vi "Periodic Tasks.vi"(8 "error in":errorcluster) -> ()   [LabVIEW 2016]
doc: "This VI runs in parallel to other tasks. It can contain as many user-defined periodic loops as you need. These can carry out PID or other sorts of timed response."
uses:
  <vilib>/Rock Robotics/WPI/Utilities/WPI_GetSetVariantRefNum.vi
  <vilib>/Rock Robotics/Network Tables/NT Write Number.vi
  <vilib>/Instr/_visa.llb/VISA Configure Serial Port (Instr).vi
  2_11_17/Systems/Global 1.vi
panel:
  out "PSI":dbl=101.0986199
  out "Drive R0 Effort":dbl format="%#_13g"
  out "Drive L0 Effort":dbl format="%#_13g"
  out "read buffer":string="B:2,X:203.00"
  in  "Search_Params":string[](array[string])=["B", "X", "Y", "W1", "H1", "W2", "H2"]
  out "Last Complete Message":string="B:2,X:203.00,Y:125.00,W1:11,H1:27,W2:8,H2:25"
  out "length":i32=44
  in  "off set":dbl format="%#_13g"
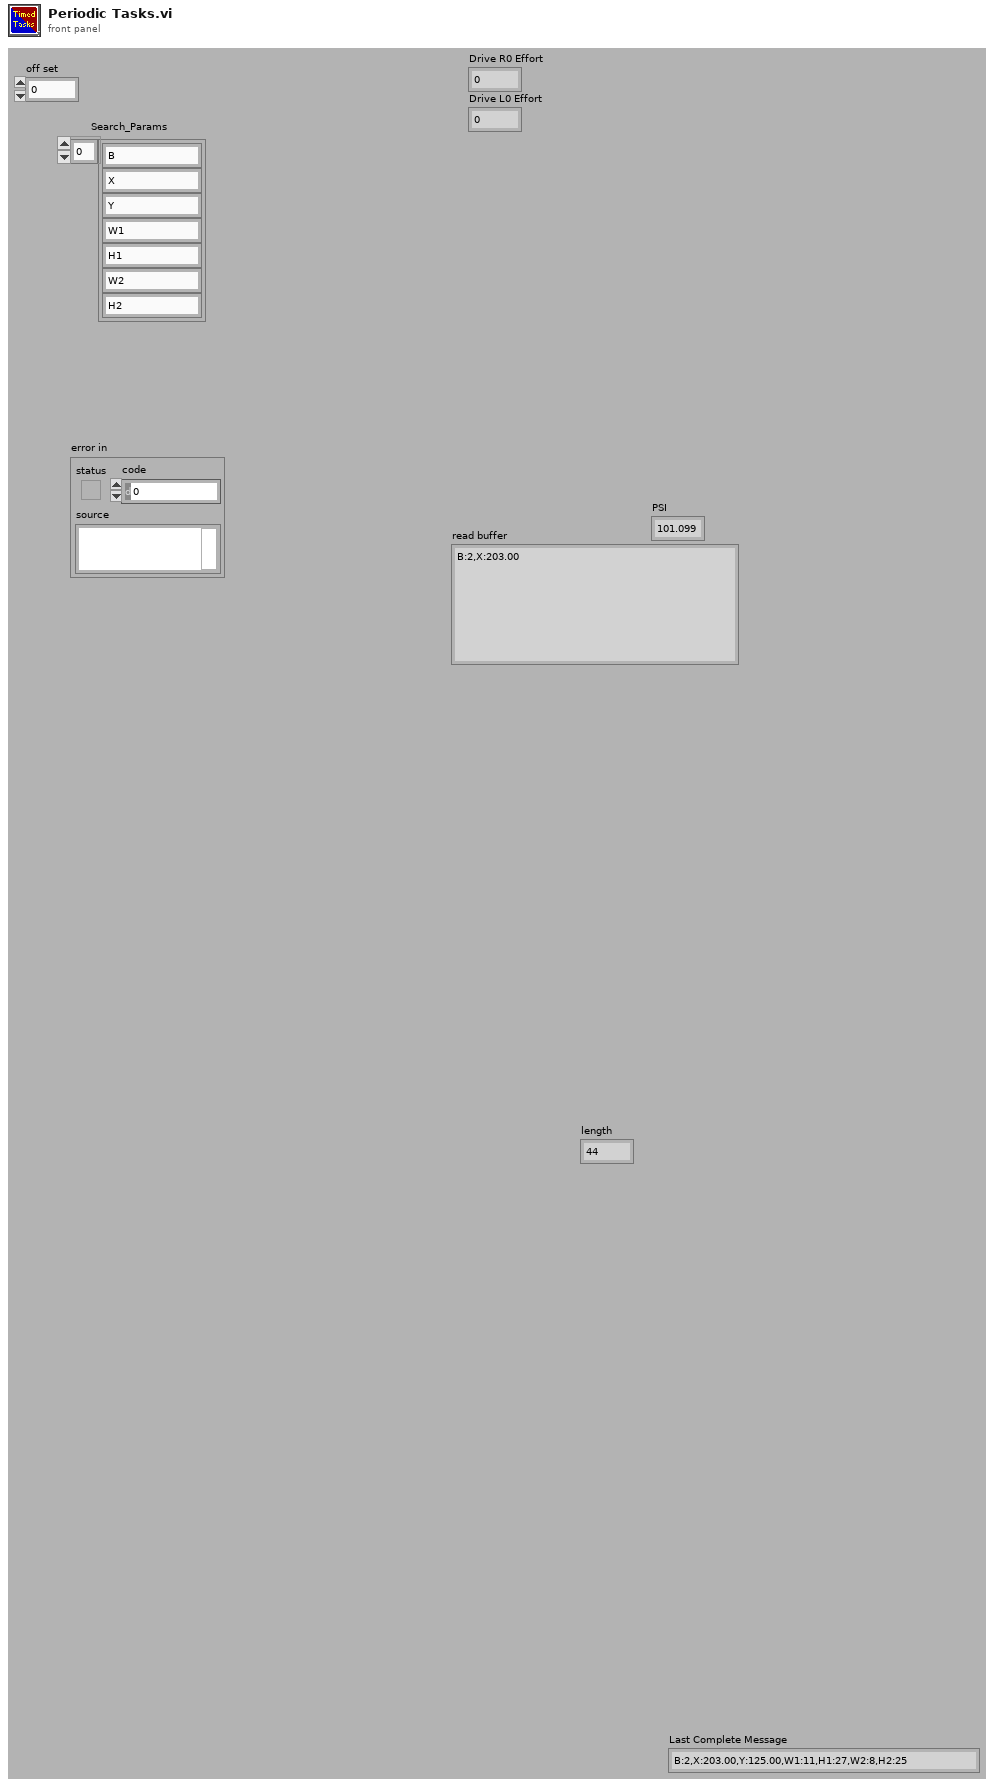
[diagram p1: front panel]
types:
  T1 = typedef "WPI_JoystickDevRef.ctl" = cluster{"Device":T2}
  T2 = typedef "WPI_JoystickDeviceEnum.ctl" = enum16{"USB 0", "USB 1", "USB 2", "USB 3", "USB 4", "USB 5"}
  T3 = typedef "WPI_AnalogChannelDevRef.ctl" = cluster{"DevStatus":errorcluster, "Analog Channel":T4}
  T4 = typedef "FPGA_AIChannel.ctl" = enum8{"AI 0", "AI 1", "AI 2", "AI 3", "AI MXP 0", "AI MXP 1", "AI MXP 2", "AI MXP 3", "Invalid"}
  T5 = typedef "WPI_MotorControlDeviceRef.ctl" = cluster{"DeviceStatus":errorcluster, "Type":T6, "PWM":cluster{"PWM Channel":T7, "DeadBand":T8}, "CAN":cluster{"Device Number":u8, "SetOutput VI Ref":variant, "GetOutput VI Ref":variant, "Enable VI Ref":variant, "Disable VI Ref":variant, "Data":variant}, "Invert":bool}
  T6 = typedef "WPI_MotorControlType.ctl" = enum16{"PWM", "CAN"}
  T7 = typedef "FPGA_DIOPWMChannel.ctl" = enum8{"PWM 0", "PWM 1", "PWM 2", "PWM 3", "PWM 4", "PWM 5", "PWM 6", "PWM 7", "PWM 8", "PWM 9", "PWM MXP 0", "PWM MXP 1", "PWM MXP 2", "PWM MXP 3", "PWM MXP 4", "PWM MXP 5", "PWM MXP 6", "PWM MXP 7", "PWM MXP 8", "PWM MXP 9", "Invalid"}
  T8 = typedef "WPI_PWMDeadband.ctl" = cluster{"Name":string, "maxPositivePwm":i32, "minPositivePwm":i32, "centerPwm":i32, "maxNegativePwm":i32, "minNegativePwm":i32, "angularRange":u16}
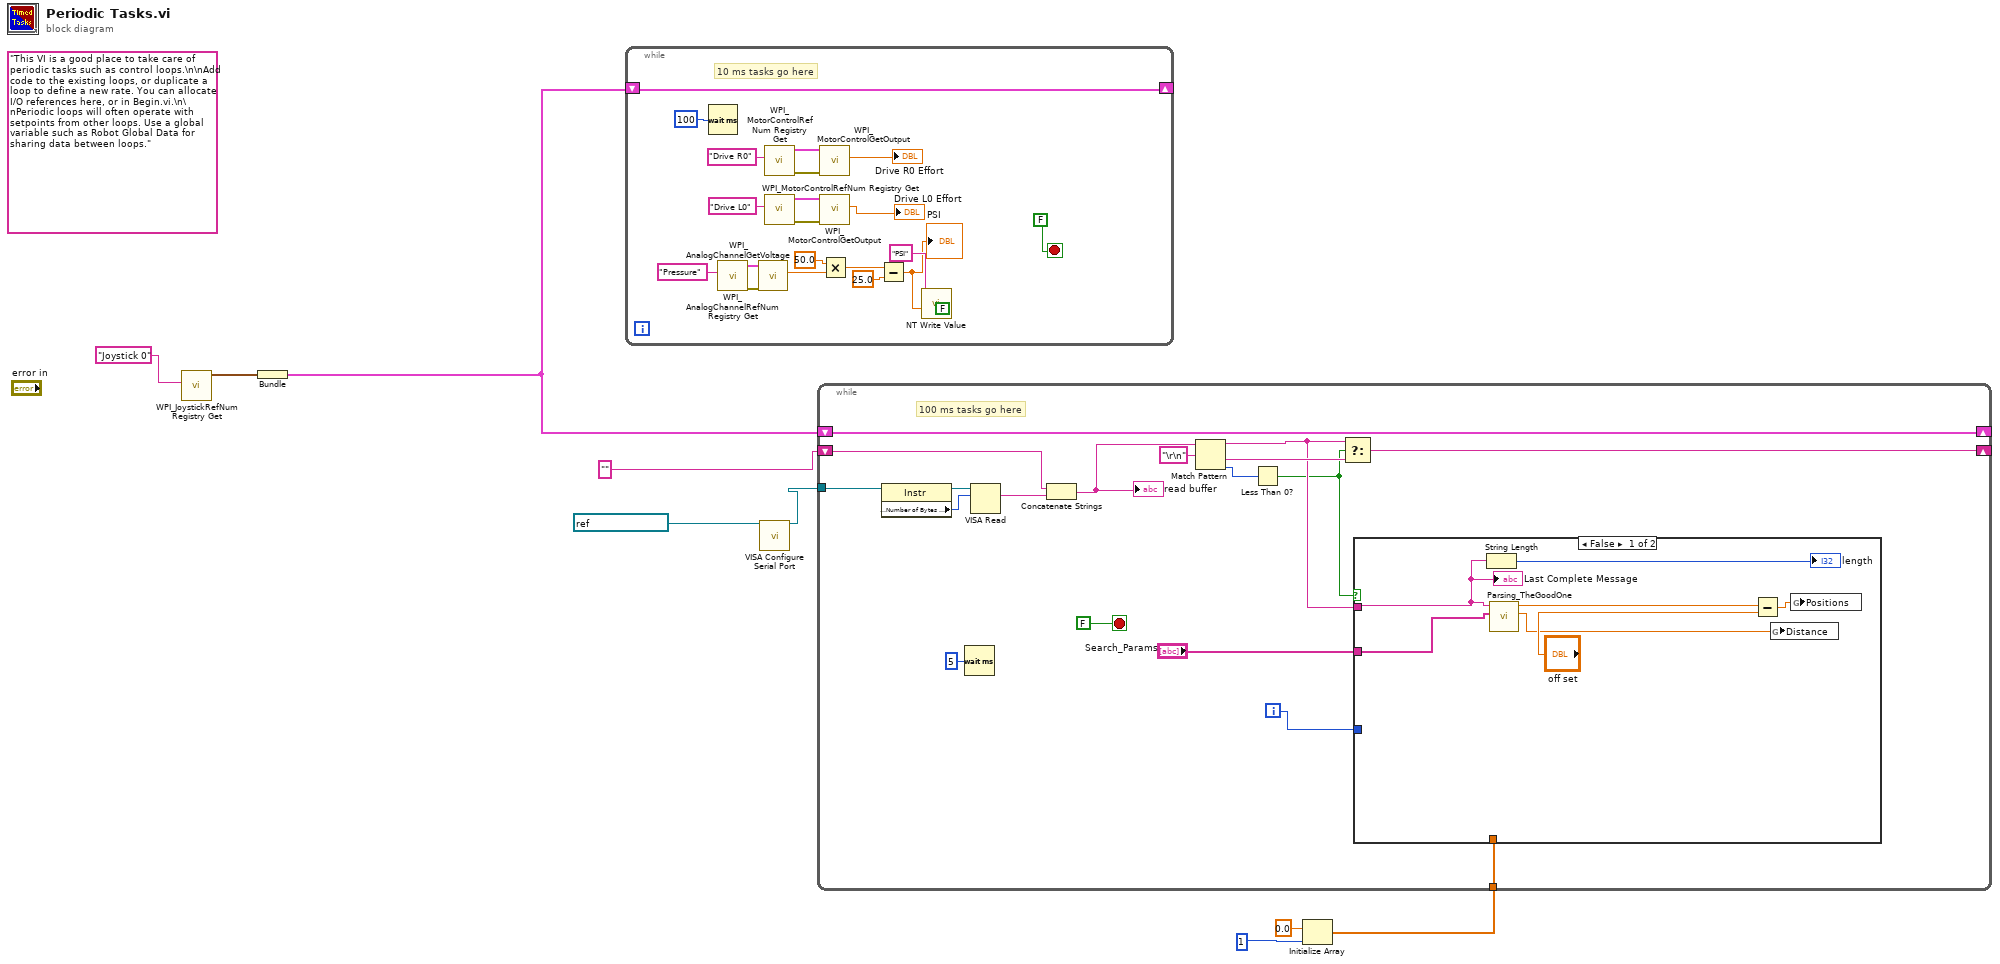
[diagram p0: block diagram]
diagram:
  (unwired) "This VI is a good place to take care of periodic tasks such as control loops.\n\nAdd code to the existing loops, or duplicate a loop to define a new rate. You can allocate I/O references here, or in Begin.vi.\n\nPeriodic loops will often operate with setpoints from other loops. Use a global variable such as Robot Global Data for sharing data between loops."
  n1 = call <vilib>:"WPI_JoystickRefNum Registry Get.vi"("refnum name"="Joystick 0") -> ("JoystickDevRef"=w2:T1)  [unwired: 1 in, 9 out]
  n2 = Bundle("JoystickDevRef"=w2) -> (w3:cluster{"JoystickDevRef":T1})  [unwired: 1 out]
  n3 = while {
    shift-right: [w27] -> _
    shift-left: w3 -> [w27]
    stop <- FALSE stop-if-true
    (unwired) FALSE
    # "10 ms tasks go here"
    n4 = Wait (ms)(milliseconds to wait=u32 100) -> ()  [unwired: 1 out]
    n5 = call <vilib>:"WPI_AnalogChannelRefNum Registry Get.vi"("refnum name"="Pressure") -> ("error out"=w18:errorcluster, "AIDeviceRef"=w17:T3)  [unwired: 9 in]
    n6 = call <vilib>:"WPI_AnalogChannelGetVoltage.vi"("error in (no error)"=w18, "AIDeviceRef"=w17) -> ("Voltage"=w15:dbl)  [unwired: 7 in, 2 out]
    n7 = call <vilib>:"WPI_MotorControlRefNum Registry Get.vi"("refnum name"="Drive R0") -> ("error out"=w22:errorcluster, "MotorControlDevRef"=w26:T5)  [unwired: 9 in]
    n8 = call <vilib>:"WPI_MotorControlRefNum Registry Get.vi"("refnum name"="Drive L0") -> ("error out"=w21:errorcluster, "MotorControlDevRef"=w23:T5)  [unwired: 9 in]
    n9 = call <vilib>:"WPI_MotorControlGetOutput.vi"("error in"=w22, "MotorControlDevRef"=w26) -> ("Output"=→"Drive R0 Effort":dbl)  [unwired: 7 in, 2 out]
    n10 = call <vilib>:"WPI_MotorControlGetOutput.vi"("error in"=w21, "MotorControlDevRef"=w23) -> ("Output"=→"Drive L0 Effort":dbl)  [unwired: 7 in, 2 out]
    n11 = Multiply(x=50.0, y=w15) -> (x*y=w13:dbl)
    n12 = Subtract(x=w13, y=25.0) -> (x-y=w10:dbl)
    "PSI" <- w10
    n13 = call-poly <vilib>:"NT Write Value.vi"("Numeric"=w10, "Name"="PSI") -> ()  [unwired: 9 in, 1 out]
  }
  n14 = call-poly "VISA Configure Serial Port"("VISA resource name"=refnum<visa-resource-name> "ASRL2::INSTR") -> ("VISA resource name out"=w5:refnum<visa-resource-name>)  [unwired: 13 in, 1 out]
  n15 = Initialize Array(0.0 ("element"), 1) -> (w9:dbl[])
  n16 = while {
    shift-right: [w46] -> _
    shift-left: w3 -> [w46]
    tunnel: w5 -> [w41]
    shift-right: [w33] -> _
    shift-left: "" -> [w40]
    tunnel: w9 -> [w30]
    i -> [w31]
    stop <- FALSE stop-if-true
    # "100 ms tasks go here"
    n17 = property class="Instr"(reference=w41) -> (reference out=w45:refnum<visa-resource-name>, "Serial Settings:Number of Bytes at Serial Port"=w44:u32)  [unwired: 1 in, 1 out]
    n18 = Wait (ms)(milliseconds to wait=u32 5) -> ()  [unwired: 1 out]
    n19 = VISA Read(VISA resource name=w45, byte count=w44) -> (read buffer=w39:string)  [unwired: 1 in, 3 out]
    n20 = Concatenate Strings(w40, w39) -> (w38:string)
    "read buffer" <- w38
    n21 = Match Pattern(string=w38, regular expression="\r\n") -> (before substring=w34:string, after substring=w35:string, offset past match=w36:i32)  [unwired: 1 in, 1 out]
    n22 = Less Than 0?(x=w36) -> (x < 0?=w32:bool)
    n23 = Select(t=w34, s=w32, f=w35) -> (s? t:f=w33:string)
    n24 = case shown="False" w32 {
      tunnel: "Search_Params" -> [w53 _]
      tunnel: w34 -> [w52 _]
      tunnel: w31 -> [_ _]
      tunnel: w30 -> [_ _]
      frame False {
        n25 = String Length(string=w52) -> (length=→"length":i32)
        n26 = call "Parsing_TheGoodOne.vi"("Search_Params"=w53, "Input"=w52) -> ("Corrected distance"=w48:dbl, "Value-Reference"=w51:dbl)  [unwired: 6 in]
        n27 = Subtract(x=w51, y="off set") -> (x-y=w49:dbl)
        n28 = global write "Global 1.vi" "Distance"(w48) -> ()
        n29 = global write "Global 1.vi" "Positions"(w49) -> ()
        "Last Complete Message" <- w52
      }
      frame True {
      }
    }
  }
